vi "E_beamline_binary_status.vi"(0 "Current State Array":bool[](array[boolean]), 2 "is safe array":bool[](array[boolean]), 3 "gv open aray":bool[](array[boolean]), 4 "manual mode array":bool[](array[boolean]), 5 "gv closed array":bool[](array[boolean])) -> (6 "index":i32, 7 "binary state":i16)   [LabVIEW 2013]
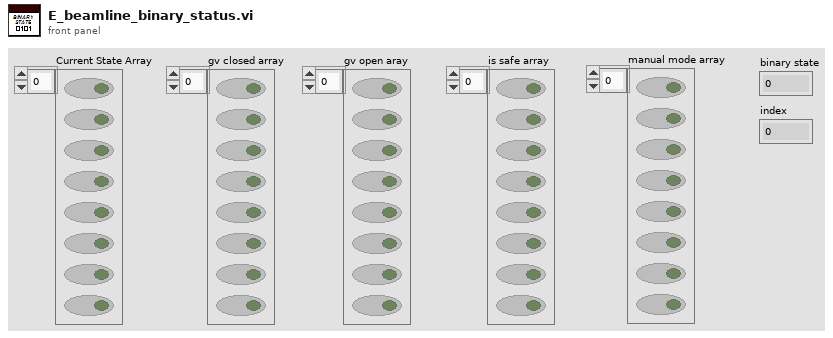
[diagram p1: front panel]
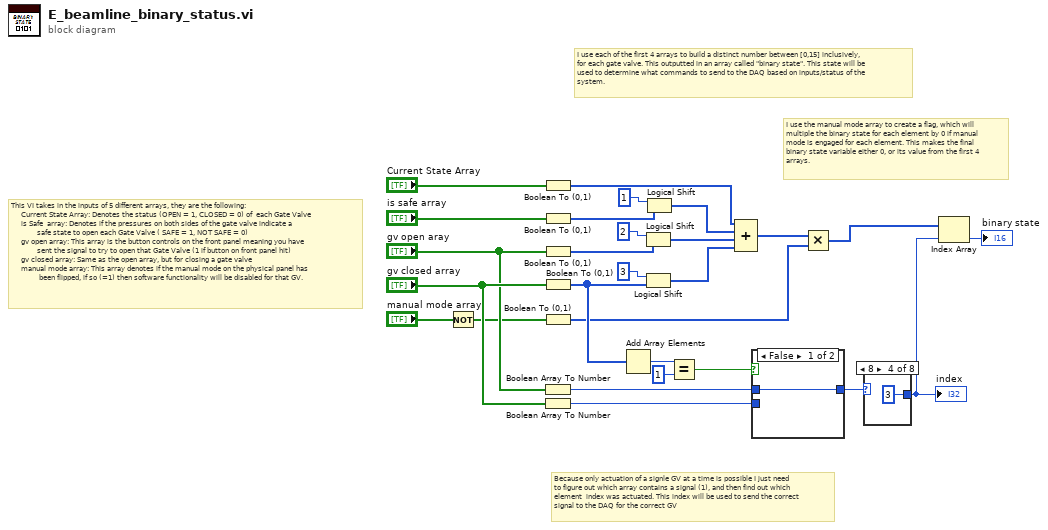
[diagram p0: block diagram]
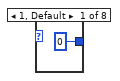
[diagram p2: hidden frame]
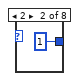
[diagram p3: hidden frame]
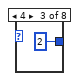
[diagram p4: hidden frame]
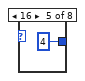
[diagram p5: hidden frame]
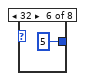
[diagram p6: hidden frame]
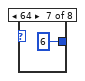
[diagram p7: hidden frame]
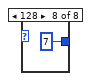
[diagram p8: hidden frame]
diagram:
  # "Because only actuation of a signle GV at a time is possible I just need\nto figure out which array contains a signal (1), and then find out which\nelement  index was actuated. This index will be used to send the correct\nsignal to the DAQ for the correct GV"
  # "I use the manual mode array to create a flag, which will\nmultiple the binary state for each element by 0 if manual\nmode is engaged for each element. This makes the final \nbinary state variable either 0, or its value from the first 4 \narrays."
  # "I use each of the first 4 arrays to build a distinct number between [0,15] inclusively, \nfor each gate valve. This outputted in an array called \"binary state\". This state will be\nused to determine what commands to send to the DAQ based on inputs/status of the\nsystem."
  # "This VI takes in the inputs of 5 different arrays, they are the following:\n     Current State Array: Denotes the status (OPEN = 1, CLOSED = 0) of  each Gate Valve\n     is Safe  array: Denotes if the pressures on both sides of the gate valve indicate a \n             safe state to open each Gate Valve ( SAFE = 1, NOT SAFE = 0) \n     gv open array: This array is the button controls on the front panel meaning you have \n             sent the signal to try to open that Gate Valve (1 if button on front panel hit)\n     gv closed array: Same as the open array, but for closing a gate valve\n     manual mode array: This array denotes if the manual mode on the physical panel has \n              been flipped, if so (=1) then software functionality will be disabled for that GV."
  n1 = Not(x="manual mode array") -> (.not. x?=w4:bool[])
  n2 = Boolean To (0,1)(Boolean="Current State Array") -> (0, 1=w16:i16[])
  n3 = Boolean To (0,1)(Boolean="is safe array") -> (0, 1=w15:i16[])
  n4 = Boolean To (0,1)(Boolean="gv open aray") -> (0, 1=w9:i16[])
  n5 = Boolean To (0,1)(Boolean="gv closed array") -> (0, 1=w12:i16[])
  n6 = Boolean To (0,1)(Boolean=w4) -> (0, 1=w2:i16[])
  n7 = Boolean Array To Number(Boolean array="gv open aray") -> (number=w6:u32)
  n8 = Boolean Array To Number(Boolean array="gv closed array") -> (number=w8:u32)
  n9 = Add Array Elements(numeric array=w12) -> (sum=w19:i16)
  n10 = Logical Shift(y=u32 2 ("x"), x=w9) -> (x << y=w26:i16[])
  n11 = Logical Shift(y=u32 3 ("x"), x=w12) -> (x << y=w25:i16[])
  n12 = Logical Shift(y=u32 1 ("x"), x=w15) -> (x << y=w27:i16[])
  n13 = Equal?(x=w19, y=i16 1) -> (x = y?=w17:bool)
  n14 = Compound Arithmetic op=ADD(w16, w27, w26, w25) -> (w3:i16[])
  n15 = case shown="False" w17 {
    tunnel: [w28 w29] -> w14
    tunnel: w8 -> [_ w29]
    tunnel: w6 -> [w28 _]
    frame False {
    }
    frame True {
    }
  }
  n16 = Multiply(x=w3, y=w2) -> (x*y=w1:i16[])
  n17 = case shown="8" w14 {
    tunnel: [0 1 2 3 4 5 6 7] -> w11
    frame 1, Default {
    }
    frame 2 {
    }
    frame 4 {
    }
    frame 8 {
    }
    frame 16 {
    }
    frame 32 {
    }
    frame 64 {
    }
    frame 128 {
    }
  }
  "index" <- w11
  n18 = Index Array(array=w1, index=w11) -> (element=→"binary state":i16)
